vi "main.vi"() -> ()   [LabVIEW 2018]
uses:
  <vilib>/Platform/TimedLoop/XDataNode/timing_clust.ctl
  <vilib>/Platform/TimedLoop/XDataNode/nitl_modes.ctl
  <vilib>/Platform/TimedLoop/XDataNode/wakeup.ctl
  <vilib>/FPGAPlugInAG/PCIe-7841R/niLvFpga_Open_PCIe-7841R.vi
  <vilib>/rvi/interface/common/dynamic/niFpgaDynamicAddResources.vi
  <vilib>/Utility/error.llb/Error Cluster From Error Code.vi
  <vilib>/rvi/errors/niLvFpgaAdjustHostInterfaceError.vi
  <vilib>/FPGAPlugInAG/Dynamic/niLvFpga_Close_Dynamic.vi
  <vilib>/rvi/interface/nirviOpenFPGA/nirviOpenFPGA.xnode
  FPGA Bitfiles/DentalRobotEther_FPGATarget_FPGA_Y1u8jArW7bo.lvbitx
  FPGA/FPGA.vi
  <vilib>/rvi/interface/nirviReadWriteControl/nirviReadWriteControl.xnode
  <vilib>/Platform/TimedLoop/XDataNode/XDataNode.xnode
  <vilib>/rvi/interface/nirviCloseFPGA/nirviCloseFPGA.xnode
  <vilib>/Platform/TimedLoop/XDataNode/XDNodeRunTimeDep.lvlib
  <vilib>/rvi/interface/Simulation/niFpgaSimulationCallBeginRW.vi
  NiFpgaLv.dll
panel:
  in  "Tab Control 2":enum32{"Setting", "OTR", "Velocity Control"}(tab)
  in  "DC":fxp<+,32,0>=0.6999999999534339
  in  "Count/revolution":i32=17408
  in  "PID":cluster{"Kp":dbl, "Kd":dbl, "Ki":dbl}={"Kp"=0.002, "Kd"=0.007, "Ki"=9e-05}
  in  "limit_mA":dbl=480.0
  in  "inverse(degree)":i32=270
  out "Voltage Detection (mV)":cluster{dbl, "limit_mA":dbl}(graph)
  in  "DIR4":bool=TRUE
  in  "OTR":bool=TRUE
  in  "Clear":bool
  out "Inverse Count":i32
  in  "Desired RPM":dbl=200.0 step=10.0 format="%.1f"
  in  "VelCtrl":bool=TRUE
  out "Finished Late_Current Feedback":u32
  out "Finished Late_Tool Control":u32
  out "Real RPM":dbl format="%.1f"
  out "store":fxp<+,32,0>[](array[numeric])
  in  "temp":i32
  in  "Inv":bool
  in  "wait":i32
  out "Position4":i32
  out "mV":i16
  in  "Rotate":bool=TRUE
  out "Finished Late_monitor":u32
  out "Finished Late_control":u32
  in  "Tab Control":enum32{"Joints", "Position"}(tab)
  in  "Joints":sgl[](array[numeric]) step=1 format="%#_6f"
  in  "Position":sgl[](array[numeric]) step=1 format="%#_6f"
  in  "Motion Control":T1
  out "Position":T2 {"Z_theta" format="%#_8f"; "Y_theta" format="%#_8f"; "X_theta" format="%#_8f"; "Z" format="%#_8f"; "Y" format="%#_8f"; "X" format="%#_8f"}
  out "Joints (degree)":T3 {"Axis 6" format="%#_8f"; "Axis 5" format="%#_8f"; "Axis 4" format="%#_8f"; "Axis 3" format="%#_8f"; "Axis 2" format="%#_8f"; "Axis 1" format="%#_8f"}
  out "Error code":u16
  out "Motion Status":T4
  in  "Robot Control":T5
  out "Robot status":T6
  in  "stop":bool
  # "Robot Arm Control"
  # "Tool Control"
  # "Monitor"
  # "Control Panel"
  # "Intermediate Informations"
  # "Tool Setting"
  # "OTR Setting"
  # "Current Feedback"
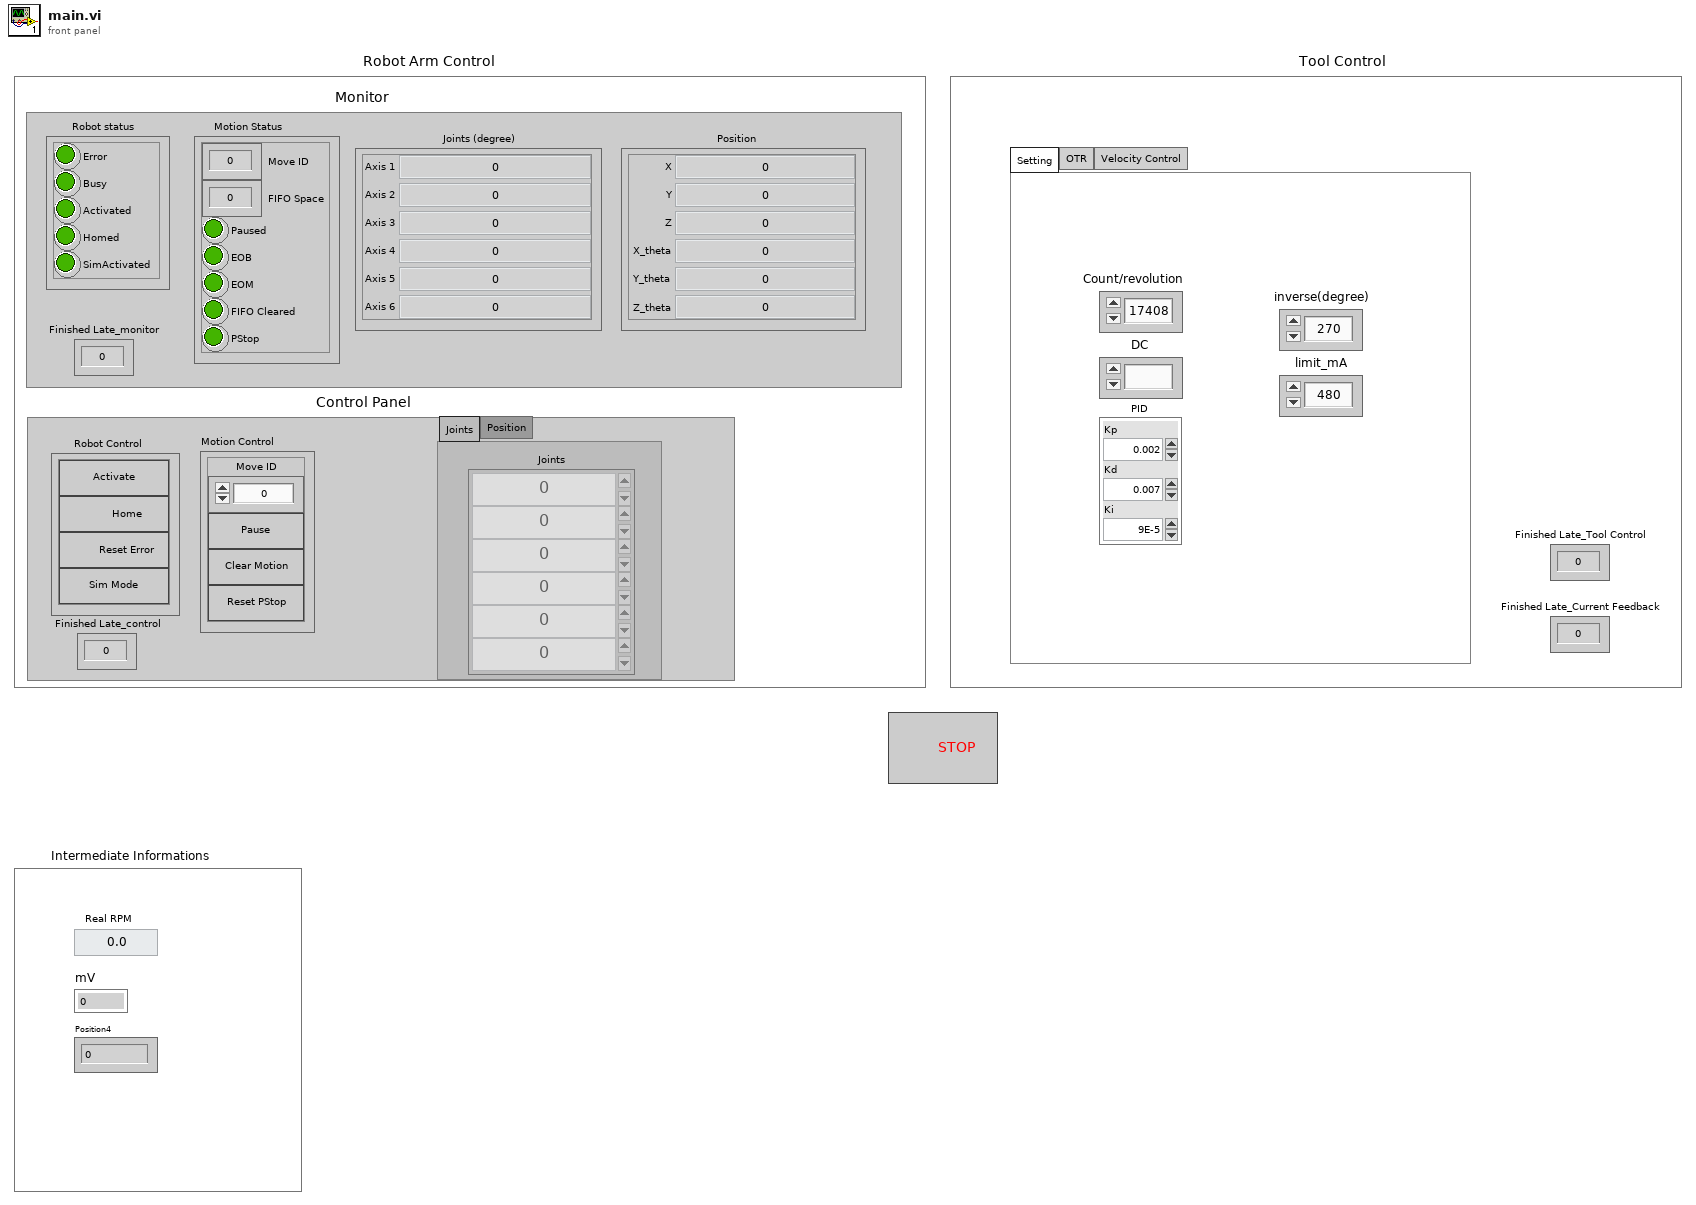
[diagram p1: front panel]
types:
  T1 = cluster{"Move ID":u16, "Pause":bool, "Clear Move":bool, "Reset PStop":bool}
  T2 = cluster{"X":sgl, "Y":sgl, "Z":sgl, "X_theta":sgl, "Y_theta":sgl, "Z_theta":sgl}
  T3 = cluster{"Axis 1":sgl, "Axis 2":sgl, "Axis 3":sgl, "Axis 4":sgl, "Axis 5":sgl, "Axis 6":sgl}
  T4 = cluster{"Move ID":dbl, "FIFO Space":dbl, "Paused":bool, "EOB":bool, "EOM":bool, "FIFO Cleared":bool, "PStop":bool}
  T5 = cluster{"Activate":bool, "Home":bool, "Reset":bool, "Sim Mode":bool}
  T6 = cluster{"Error":bool, "Busy":bool, "Activated":bool, "Homed":bool, "SimActivated":bool}
  T7 = typedef "XDNodeRunTimeDep.lvlib/timing_clust.ctl" = cluster{"Expected End [f-1]":u64, "Actual End [f-1]":u64, "Finished Late? [f-1]":bool, "Expected End [i-1]":u64, "Actual End [i-1]":u64, "Finished Late? [i-1]":bool, "Expected Start [i]":u64, "Actual Start [i]":u64, "Expected Start [f]":u64, "Actual Start [f]":u64, "Source Name":string, "Structure Name":string, "Period":i64, "Deadline":i64, "Offset":i64, "Start":i64, "Priority":i32, "Timeout":i32, "Mode":T8, "Wakeup Reason":T9, "Error":errorcluster, "Source Type":string, "Secondary Source Type":string, "Global End Time":u64, "Global Start Time":u64, "Frame Duration":u64, "Iteration Duration":u64, "Assigned CPU":i32, "I/O Scan Engine Mode":u32}
  T8 = typedef "XDNodeRunTimeDep.lvlib/nitl_modes.ctl" = enum32{"No Change", "Process missed periods, maintain original phase", "Discard missed periods, maintain original phase", "Process missed periods, ignore original phase", "Discard missed periods, ignore original phase"}
  T9 = typedef "XDNodeRunTimeDep.lvlib/wakeup.ctl" = enum32{"Normal", "Aborted", "Asynchronous wakeup", "Timing source error", "Timed loop error", "Timeout"}
  T10 = cluster{"Connector0/AI0":i16, "Connector0/AI1":i16, "Connector0/AI2":i16, "Connector0/AI3":i16, "Connector0/AI4":i16}
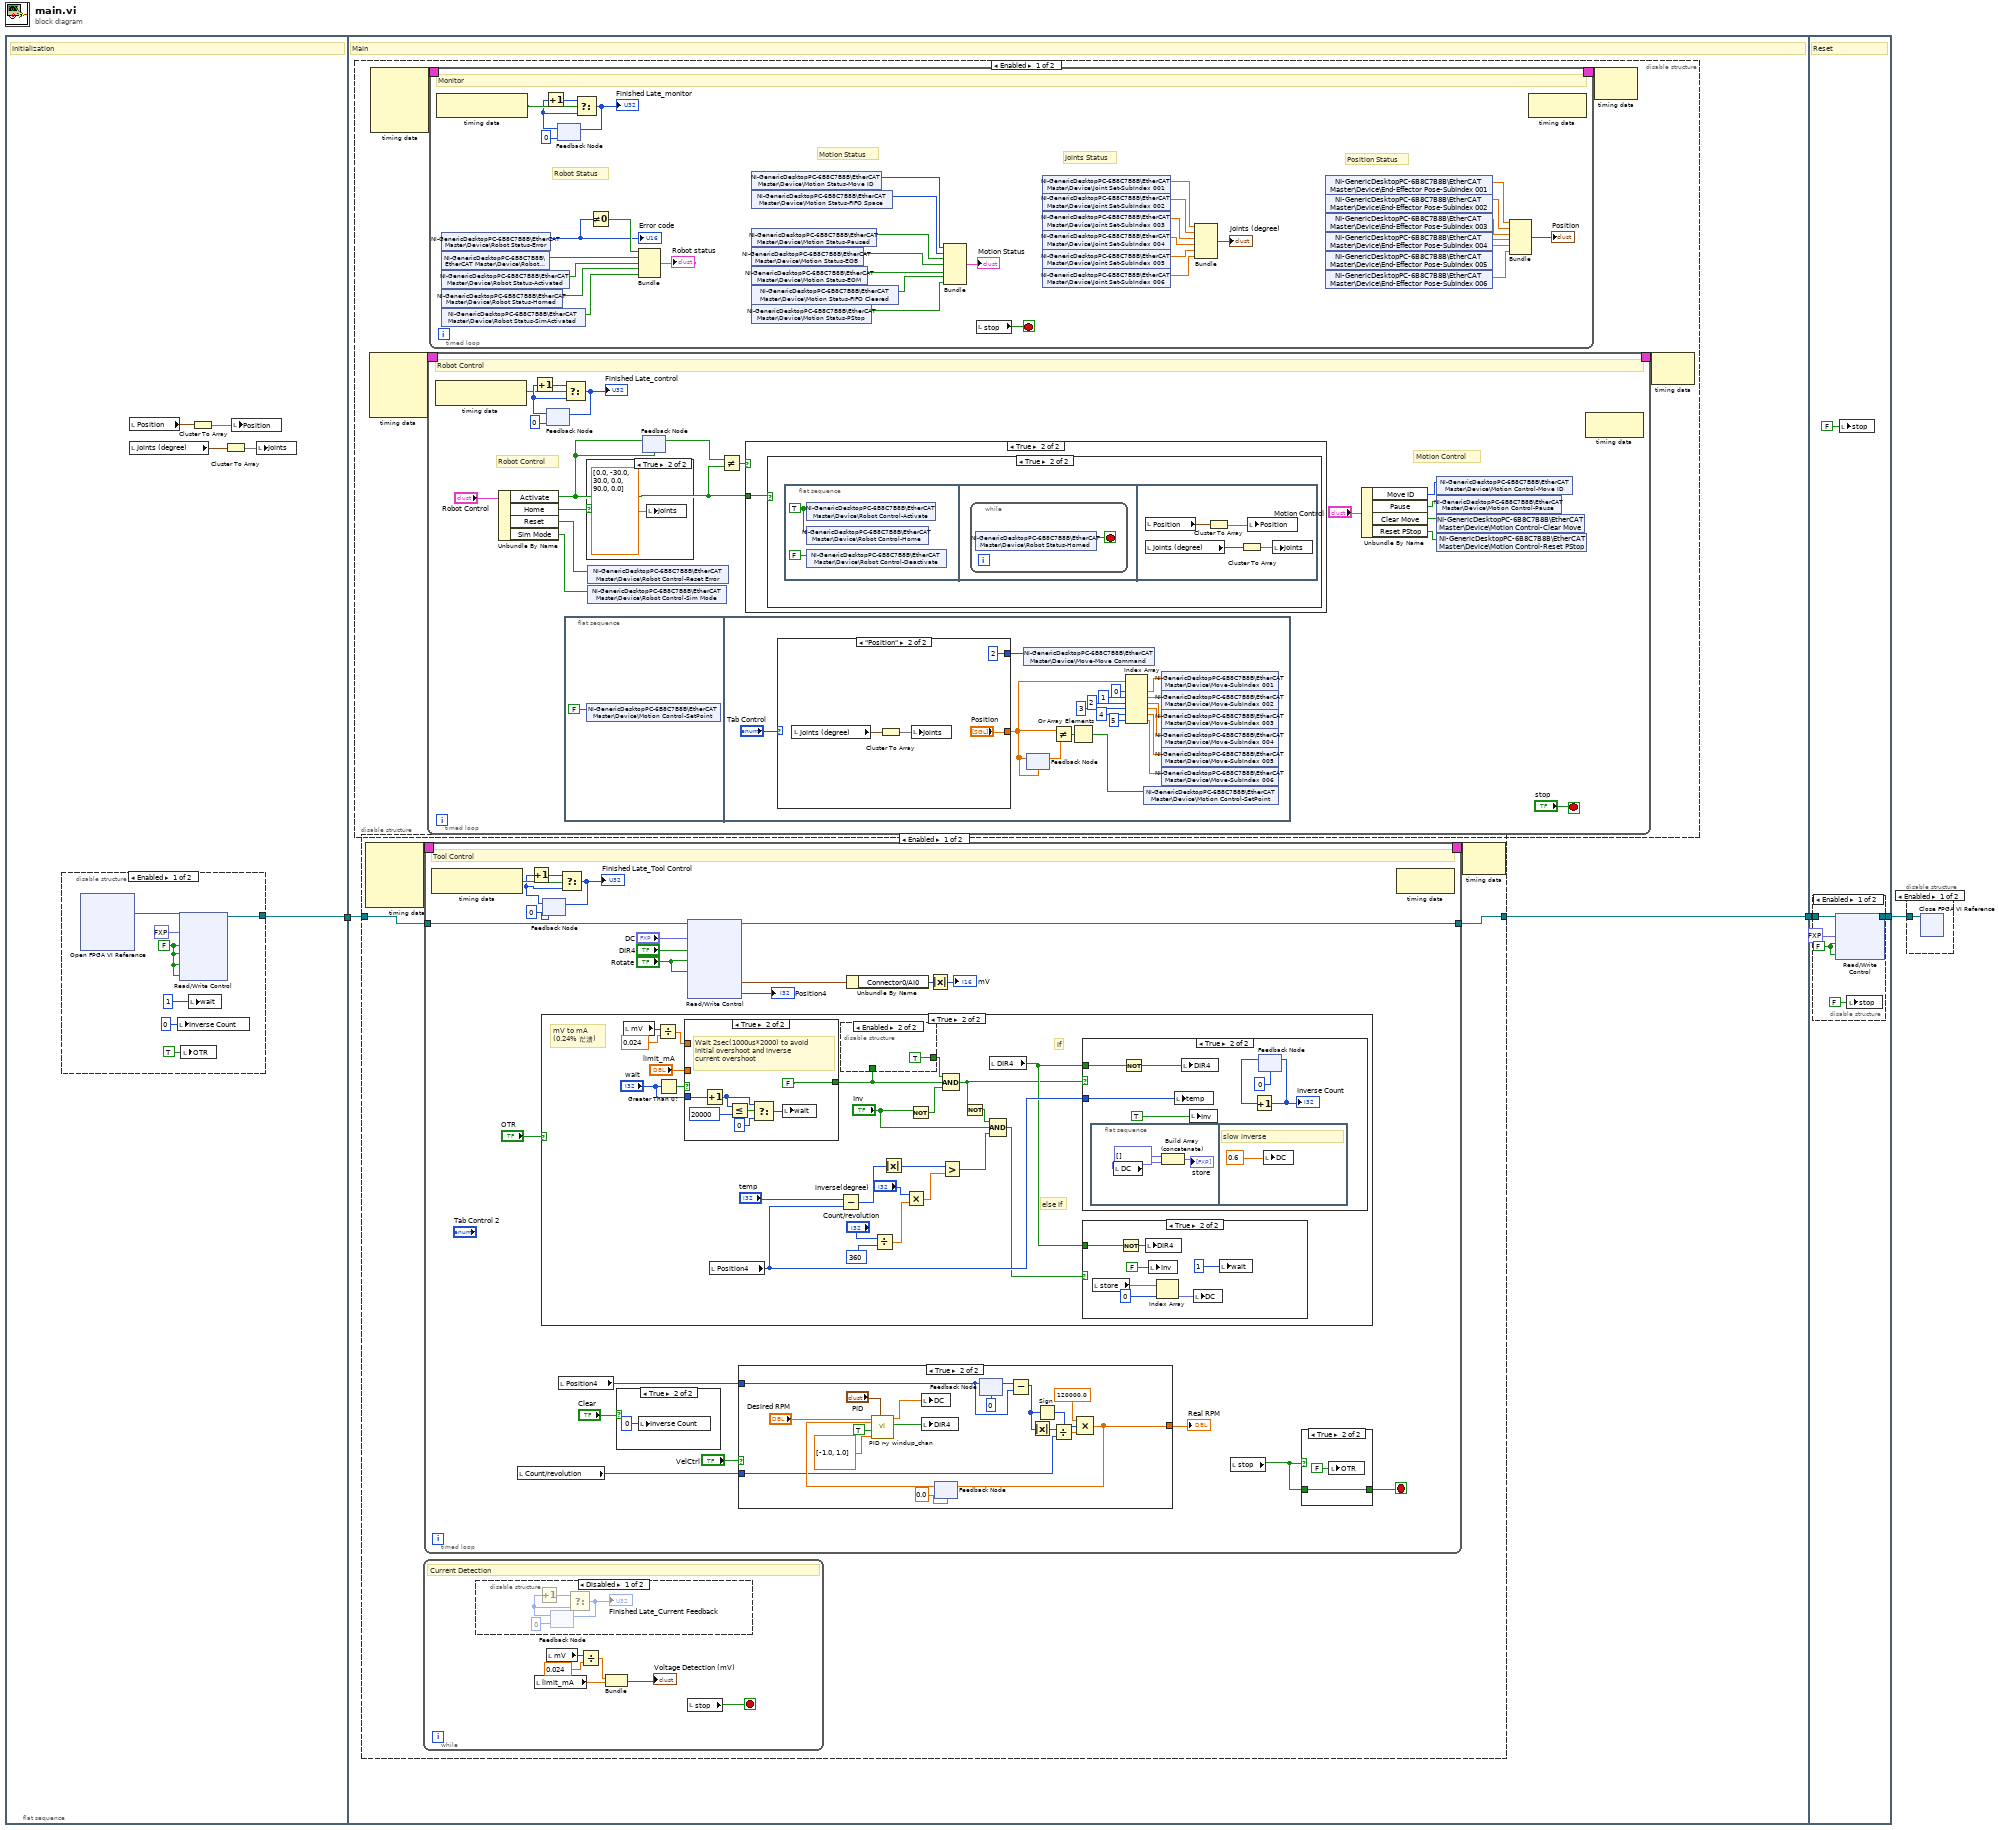
[diagram p0: block diagram]
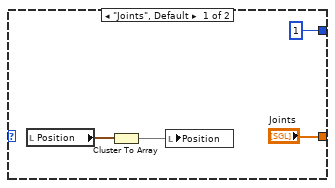
[diagram p4: hidden frame]
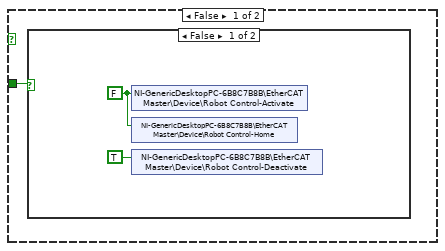
[diagram p5: hidden frame]
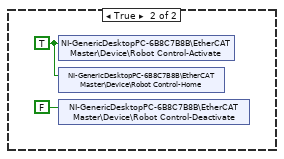
[diagram p6: hidden frame]
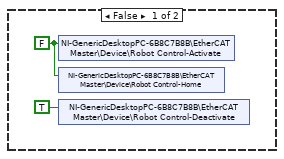
[diagram p7: hidden frame]
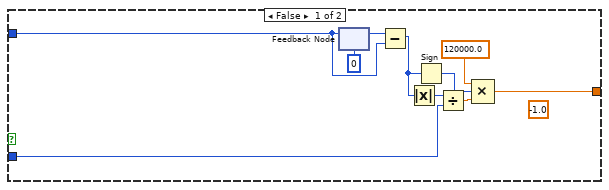
[diagram p13: hidden frame]
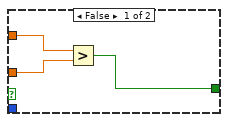
[diagram p15: hidden frame]
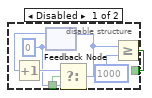
[diagram p16: hidden frame]
diagram:
  n1 = flat-sequence {
    tunnel: [w8] -> w3
    tunnel: w3 -> [w17]
    tunnel: [w16] -> w2
    tunnel: w2 -> [w263]
    tunnel: [w262] -> w1
    frame #0 {
      # "Initialization"
      n2 = disable-structure shown="Enabled" {
        disable-tunnel: [w15 _] -> w8
        frame Enabled {
          w13 = FALSE ("Reset4")
          n3 = xnode "Open FPGA VI Reference"() -> ("FPGA VI Reference Out"=w9:refnum<k20>)  [unwired: 2 in, 1 out]
          n4 = local write "Inverse Count"(0 ("Inverse Count")) -> ()
          n5 = xnode "Read/Write Control"("FPGA VI Reference In"=w9, "CH4 DC"=fxp<+,32,0> 0.0, "Reset4"=w13, "STBY4"=w13, "ENA4"=w13, "DIR4"=w13) -> ("FPGA VI Reference Out"=w15:refnum<k20>)  [unwired: 1 in, 1 out]
          n6 = local write "OTR"(TRUE ("OTR")) -> ()
          n7 = local write "wait"(1 ("wait")) -> ()
        }
        frame Disabled {
        }
      }
      n8 = local read "Position"() -> (w6:T2)
      n9 = local read "Joints (degree)"() -> (w4:T3)
      n10 = Cluster To Array(cluster=w6) -> (array=w7:sgl[])
      n11 = Cluster To Array(cluster=w4) -> (array=w5:sgl[])
      n12 = local write "Position"(w7) -> ()
      n13 = local write "Joints"(w5) -> ()
    }
    frame #1 {
      # "Main"
      n14 = disable-structure shown="Enabled" {
        frame Enabled {
          n15 = node-c288() -> (w21:T7)  [unwired: 4 in]
          n16 = node-c288() -> (w19:T7)  [unwired: 4 in]
          n17 = timed-loop {
            timing: w21 -> [_]
            timing-out: [_] -> w20
            stop <- "stop" stop-if-true
            # "Motion Control"
            # "Robot Control"
            # "Robot Control"
            n18 = node-c288() -> (w66:bool)  [unwired: 1 in]
            n19 = Unbundle By Name("Robot Control") -> ("Activate"=w63:bool, "Home"=w77:bool, "Reset"=w76:bool, "Sim Mode"=w75:bool)
            n20 = feedback #1(u32 0) -> (w68:u32)
            n21 = Increment(x=w68) -> (x+1=w69:u32)
            n22 = Select(t=w69, s=w66, f=w68) -> (s? t:f=w65:u32)
            "Finished Late_control" <- w65
            n23 = feedback-in #1(w65) -> ()
            n24 = flat-sequence {
              frame #0 {
                n25 = shared-variable "NI-GenericDesktopPC-6B8C7B8B\\EtherCAT Master\\Device\\Motion Control-SetPoint"(FALSE ("Motion Control-SetPoint")) -> ()  [unwired: 1 in, 1 out]
              }
              frame #1 {
                n26 = case shown="\"Position\"" "Tab Control" {
                  tunnel: [u32 1 ("Move-Move Command") u32 2 ("Move-Move Command")] -> w88
                  tunnel: ["Joints" "Position"] -> w87
                  frame "Joints", Default {
                    n27 = local read "Position"() -> (w100:T2)
                    n28 = Cluster To Array(cluster=w100) -> (array=w99:sgl[])
                    n29 = local write "Position"(w99) -> ()
                  }
                  frame "Position" {
                    n30 = local read "Joints (degree)"() -> (w105:T3)
                    n31 = Cluster To Array(cluster=w105) -> (array=w104:sgl[])
                    n32 = local write "Joints"(w104) -> ()
                  }
                }
                n33 = shared-variable "NI-GenericDesktopPC-6B8C7B8B\\EtherCAT Master\\Device\\Move-Move Command"(w88) -> ()  [unwired: 1 in, 1 out]
                n34 = feedback #2(w87) -> (w98:sgl[])
                n35 = feedback-in #2(w87) -> ()
                n36 = Not Equal?(x=w87, y=w98) -> (x != y?=w97:bool[])
                n37 = Or Array Elements(Boolean array=w97) -> (logical OR=w90:bool)
                n38 = Index Array(array=w87, index #1=0 ("index"), index #2=1 ("index"), index #3=2 ("index"), index #4=3 ("index"), index #5=4 ("index"), index #6=5 ("index")) -> (element #1=w86:sgl, element #2=w85:sgl, element #3=w84:sgl, element #4=w83:sgl, element #5=w82:sgl, element #6=w81:sgl)
                n39 = shared-variable "NI-GenericDesktopPC-6B8C7B8B\\EtherCAT Master\\Device\\Motion Control-SetPoint"(w90) -> ()  [unwired: 1 in, 1 out]
                n40 = shared-variable "NI-GenericDesktopPC-6B8C7B8B\\EtherCAT Master\\Device\\Move-SubIndex 001"(w86) -> ()  [unwired: 1 in, 1 out]
                n41 = shared-variable "NI-GenericDesktopPC-6B8C7B8B\\EtherCAT Master\\Device\\Move-SubIndex 002"(w85) -> ()  [unwired: 1 in, 1 out]
                n42 = shared-variable "NI-GenericDesktopPC-6B8C7B8B\\EtherCAT Master\\Device\\Move-SubIndex 003"(w84) -> ()  [unwired: 1 in, 1 out]
                n43 = shared-variable "NI-GenericDesktopPC-6B8C7B8B\\EtherCAT Master\\Device\\Move-SubIndex 004"(w83) -> ()  [unwired: 1 in, 1 out]
                n44 = shared-variable "NI-GenericDesktopPC-6B8C7B8B\\EtherCAT Master\\Device\\Move-SubIndex 005"(w82) -> ()  [unwired: 1 in, 1 out]
                n45 = shared-variable "NI-GenericDesktopPC-6B8C7B8B\\EtherCAT Master\\Device\\Move-SubIndex 006"(w81) -> ()  [unwired: 1 in, 1 out]
              }
            }
            n46 = case shown="True" w77 {
              frame False {
              }
              frame True {
                n47 = local write "Joints"(sgl[] [0.0, -30.0, 30.0, 0.0, 90.0, 0.0] ("Move SubIndex")) -> ()
              }
            }
            n48 = shared-variable "NI-GenericDesktopPC-6B8C7B8B\\EtherCAT Master\\Device\\Robot Control-Reset Error"(w76) -> ()  [unwired: 1 in, 1 out]
            n49 = shared-variable "NI-GenericDesktopPC-6B8C7B8B\\EtherCAT Master\\Device\\Robot Control-Sim Mode"(w75) -> ()  [unwired: 1 in, 1 out]
            n50 = feedback-in #3(w63) -> ()
            n51 = feedback #3(w63) -> (w62:bool)
            n52 = Not Equal?(x=w62, y=w63) -> (x != y?=w64:bool)
            n53 = case shown="True" w64 {
              tunnel: w63 -> [w107 w112]
              frame False {
                n54 = case shown="False" w107 {
                  frame False {
                    w108 = FALSE ("Robot Control-Activate")
                    n55 = shared-variable "NI-GenericDesktopPC-6B8C7B8B\\EtherCAT Master\\Device\\Robot Control-Activate"(w108) -> ()  [unwired: 1 in, 1 out]
                    n56 = shared-variable "NI-GenericDesktopPC-6B8C7B8B\\EtherCAT Master\\Device\\Robot Control-Home"(w108) -> ()  [unwired: 1 in, 1 out]
                    n57 = shared-variable "NI-GenericDesktopPC-6B8C7B8B\\EtherCAT Master\\Device\\Robot Control-Deactivate"(TRUE ("Robot Control-Deactivate")) -> ()  [unwired: 1 in, 1 out]
                  }
                  frame True {
                    w111 = TRUE ("Robot Control-Activate")
                    n58 = shared-variable "NI-GenericDesktopPC-6B8C7B8B\\EtherCAT Master\\Device\\Robot Control-Activate"(w111) -> ()  [unwired: 1 in, 1 out]
                    n59 = shared-variable "NI-GenericDesktopPC-6B8C7B8B\\EtherCAT Master\\Device\\Robot Control-Home"(w111) -> ()  [unwired: 1 in, 1 out]
                    n60 = shared-variable "NI-GenericDesktopPC-6B8C7B8B\\EtherCAT Master\\Device\\Robot Control-Deactivate"(FALSE ("Robot Control-Deactivate")) -> ()  [unwired: 1 in, 1 out]
                  }
                }
              }
              frame True {
                n61 = case shown="True" w112 {
                  frame False {
                    w114 = FALSE ("Robot Control-Activate")
                    n62 = shared-variable "NI-GenericDesktopPC-6B8C7B8B\\EtherCAT Master\\Device\\Robot Control-Activate"(w114) -> ()  [unwired: 1 in, 1 out]
                    n63 = shared-variable "NI-GenericDesktopPC-6B8C7B8B\\EtherCAT Master\\Device\\Robot Control-Home"(w114) -> ()  [unwired: 1 in, 1 out]
                    n64 = shared-variable "NI-GenericDesktopPC-6B8C7B8B\\EtherCAT Master\\Device\\Robot Control-Deactivate"(TRUE ("Robot Control-Deactivate")) -> ()  [unwired: 1 in, 1 out]
                  }
                  frame True {
                    n65 = flat-sequence {
                      frame #0 {
                        w116 = TRUE ("Robot Control-Activate")
                        n66 = shared-variable "NI-GenericDesktopPC-6B8C7B8B\\EtherCAT Master\\Device\\Robot Control-Activate"(w116) -> ()  [unwired: 1 in, 1 out]
                        n67 = shared-variable "NI-GenericDesktopPC-6B8C7B8B\\EtherCAT Master\\Device\\Robot Control-Home"(w116) -> ()  [unwired: 1 in, 1 out]
                        n68 = shared-variable "NI-GenericDesktopPC-6B8C7B8B\\EtherCAT Master\\Device\\Robot Control-Deactivate"(FALSE ("Robot Control-Deactivate")) -> ()  [unwired: 1 in, 1 out]
                      }
                      frame #1 {
                        n69 = while {
                          stop <- w117 stop-if-true
                          n70 = shared-variable "NI-GenericDesktopPC-6B8C7B8B\\EtherCAT Master\\Device\\Robot Status-Homed"() -> (w117:bool)  [unwired: 1 in, 1 out]
                        }
                      }
                      frame #2 {
                        n71 = local read "Position"() -> (w119:T2)
                        n72 = local read "Joints (degree)"() -> (w121:T3)
                        n73 = Cluster To Array(cluster=w119) -> (array=w118:sgl[])
                        n74 = Cluster To Array(cluster=w121) -> (array=w120:sgl[])
                        n75 = local write "Position"(w118) -> ()
                        n76 = local write "Joints"(w120) -> ()
                      }
                    }
                  }
                }
              }
            }
            n77 = Unbundle By Name("Motion Control") -> ("Move ID"=w73:u16, "Pause"=w72:bool, "Clear Move"=w71:bool, "Reset PStop"=w70:bool)
            n78 = shared-variable "NI-GenericDesktopPC-6B8C7B8B\\EtherCAT Master\\Device\\Motion Control-Move ID"(w73) -> ()  [unwired: 1 in, 1 out]
            n79 = shared-variable "NI-GenericDesktopPC-6B8C7B8B\\EtherCAT Master\\Device\\Motion Control-Pause"(w72) -> ()  [unwired: 1 in, 1 out]
            n80 = shared-variable "NI-GenericDesktopPC-6B8C7B8B\\EtherCAT Master\\Device\\Motion Control-Clear Move"(w71) -> ()  [unwired: 1 in, 1 out]
            n81 = shared-variable "NI-GenericDesktopPC-6B8C7B8B\\EtherCAT Master\\Device\\Motion Control-Reset PStop"(w70) -> ()  [unwired: 1 in, 1 out]
            n82 = node-c288() -> ()  [unwired: 1 in, 1 out]
          }
          n83 = timed-loop {
            timing: w19 -> [_]
            timing-out: [_] -> w18
            stop <- w44 stop-if-true
            # "Position Status"
            # "Joints Status"
            # "Motion Status"
            # "Robot Status"
            # "Monitor"
            n84 = node-c288() -> (w46:bool)  [unwired: 1 in]
            n85 = shared-variable "NI-GenericDesktopPC-6B8C7B8B\\EtherCAT Master\\Device\\Robot Status-Error"() -> (w55:u16)  [unwired: 1 in, 1 out]
            "Error code" <- w55
            n86 = shared-variable "NI-GenericDesktopPC-6B8C7B8B\\EtherCAT Master\\Device\\Robot Status-Busy"() -> (w50:bool)  [unwired: 1 in, 1 out]
            n87 = shared-variable "NI-GenericDesktopPC-6B8C7B8B\\EtherCAT Master\\Device\\Robot Status-Activated"() -> (w51:bool)  [unwired: 1 in, 1 out]
            n88 = shared-variable "NI-GenericDesktopPC-6B8C7B8B\\EtherCAT Master\\Device\\Robot Status-Homed"() -> (w52:bool)  [unwired: 1 in, 1 out]
            n89 = shared-variable "NI-GenericDesktopPC-6B8C7B8B\\EtherCAT Master\\Device\\Robot Status-SimActivated"() -> (w53:bool)  [unwired: 1 in, 1 out]
            n90 = feedback #4(u32 0) -> (w45:u32)
            n91 = Increment(x=w45) -> (x+1=w49:u32)
            n92 = Select(t=w49, s=w46, f=w45) -> (s? t:f=w47:u32)
            "Finished Late_monitor" <- w47
            n93 = feedback-in #4(w47) -> ()
            n94 = Not Equal To 0?(x=w55) -> (x != 0?=w56:bool)
            n95 = Bundle(w56, w50, w51, w52, w53) -> (→"Robot status":cluster{bool, bool, bool, bool, bool})  [unwired: 1 in]
            n96 = shared-variable "NI-GenericDesktopPC-6B8C7B8B\\EtherCAT Master\\Device\\Motion Status-Move ID"() -> (w36:u16)  [unwired: 1 in, 1 out]
            n97 = shared-variable "NI-GenericDesktopPC-6B8C7B8B\\EtherCAT Master\\Device\\Motion Status-FIFO Space"() -> (w37:u16)  [unwired: 1 in, 1 out]
            n98 = shared-variable "NI-GenericDesktopPC-6B8C7B8B\\EtherCAT Master\\Device\\Motion Status-Paused"() -> (w38:bool)  [unwired: 1 in, 1 out]
            n99 = shared-variable "NI-GenericDesktopPC-6B8C7B8B\\EtherCAT Master\\Device\\Motion Status-EOB"() -> (w39:bool)  [unwired: 1 in, 1 out]
            n100 = shared-variable "NI-GenericDesktopPC-6B8C7B8B\\EtherCAT Master\\Device\\Motion Status-EOM"() -> (w40:bool)  [unwired: 1 in, 1 out]
            n101 = shared-variable "NI-GenericDesktopPC-6B8C7B8B\\EtherCAT Master\\Device\\Motion Status-FIFO Cleared"() -> (w41:bool)  [unwired: 1 in, 1 out]
            n102 = shared-variable "NI-GenericDesktopPC-6B8C7B8B\\EtherCAT Master\\Device\\Motion Status-PStop"() -> (w42:bool)  [unwired: 1 in, 1 out]
            n103 = Bundle(w36, w37, w38, w39, w40, w41, w42) -> (→"Motion Status":cluster{u16, u16, bool, bool, bool, bool, bool})  [unwired: 1 in]
            n104 = local read "stop"() -> (w44:bool)
            n105 = shared-variable "NI-GenericDesktopPC-6B8C7B8B\\EtherCAT Master\\Device\\Joint Set-SubIndex 001"() -> (w22:sgl)  [unwired: 1 in, 1 out]
            n106 = shared-variable "NI-GenericDesktopPC-6B8C7B8B\\EtherCAT Master\\Device\\Joint Set-SubIndex 002"() -> (w23:sgl)  [unwired: 1 in, 1 out]
            n107 = shared-variable "NI-GenericDesktopPC-6B8C7B8B\\EtherCAT Master\\Device\\Joint Set-SubIndex 003"() -> (w24:sgl)  [unwired: 1 in, 1 out]
            n108 = shared-variable "NI-GenericDesktopPC-6B8C7B8B\\EtherCAT Master\\Device\\Joint Set-SubIndex 004"() -> (w25:sgl)  [unwired: 1 in, 1 out]
            n109 = shared-variable "NI-GenericDesktopPC-6B8C7B8B\\EtherCAT Master\\Device\\Joint Set-SubIndex 005"() -> (w26:sgl)  [unwired: 1 in, 1 out]
            n110 = shared-variable "NI-GenericDesktopPC-6B8C7B8B\\EtherCAT Master\\Device\\Joint Set-SubIndex 006"() -> (w27:sgl)  [unwired: 1 in, 1 out]
            n111 = Bundle(w22, w23, w24, w25, w26, w27) -> (→"Joints (degree)":cluster{sgl, sgl, sgl, sgl, sgl, sgl})  [unwired: 1 in]
            n112 = shared-variable "NI-GenericDesktopPC-6B8C7B8B\\EtherCAT Master\\Device\\End-Effector Pose-SubIndex 001"() -> (w29:sgl)  [unwired: 1 in, 1 out]
            n113 = shared-variable "NI-GenericDesktopPC-6B8C7B8B\\EtherCAT Master\\Device\\End-Effector Pose-SubIndex 002"() -> (w30:sgl)  [unwired: 1 in, 1 out]
            n114 = shared-variable "NI-GenericDesktopPC-6B8C7B8B\\EtherCAT Master\\Device\\End-Effector Pose-SubIndex 003"() -> (w31:sgl)  [unwired: 1 in, 1 out]
            n115 = shared-variable "NI-GenericDesktopPC-6B8C7B8B\\EtherCAT Master\\Device\\End-Effector Pose-SubIndex 004"() -> (w32:sgl)  [unwired: 1 in, 1 out]
            n116 = shared-variable "NI-GenericDesktopPC-6B8C7B8B\\EtherCAT Master\\Device\\End-Effector Pose-SubIndex 005"() -> (w33:sgl)  [unwired: 1 in, 1 out]
            n117 = shared-variable "NI-GenericDesktopPC-6B8C7B8B\\EtherCAT Master\\Device\\End-Effector Pose-SubIndex 006"() -> (w34:sgl)  [unwired: 1 in, 1 out]
            n118 = Bundle(w29, w30, w31, w32, w33, w34) -> (→"Position":cluster{sgl, sgl, sgl, sgl, sgl, sgl})  [unwired: 1 in]
            n119 = node-c288() -> ()  [unwired: 1 in, 1 out]
          }
          n120 = node-c288(w18) -> ()  [unwired: 1 out]
          n121 = node-c288(w20) -> ()  [unwired: 1 out]
        }
        frame Disabled {
        }
      }
      n122 = disable-structure shown="Enabled" {
        disable-tunnel: w17 -> [w129 _]
        disable-tunnel: [w128 _] -> w16
        frame Enabled {
          n123 = node-c288() -> (w131:T7)  [unwired: 4 in]
          n124 = while {
            stop <- w135 stop-if-true
            # "Current Detection"
            n125 = disable-structure shown="Disabled" {
              frame Disabled {
                n126 = feedback #5(u32 0) -> (w142:u32)
                n127 = Increment(x=w142) -> (x+1=w141:u32)
                n128 = Select(t=w141, f=w142) -> (s=w139:bool, s? t:f=w140:u32)
                "Finished Late_Current Feedback" <- w140
                n129 = feedback-in #5(w140) -> ()
              }
              frame Enabled {
              }
            }
            n130 = local read "limit_mA"() -> (w133:dbl)
            n131 = local read "mV"() -> (w136:i16)
            n132 = Divide(x=w136, y=0.024) -> (x/y=w134:dbl)
            n133 = Bundle(w134, "limit_mA"=w133) -> (→"Voltage Detection (mV)":cluster{dbl, "limit_mA":dbl})  [unwired: 1 in]
            n134 = local read "stop"() -> (w135:bool)
          }
          n135 = timed-loop {
            timing: w131 -> [_]
            timing-out: [_] -> w130
            tunnel: w129 -> [w164]
            tunnel: [w143] -> w128
            stop <- w154 stop-if-true
            # "Tool Control"
            n136 = node-c288() -> (w147:bool)  [unwired: 1 in]
            n137 = local read "Count/revolution"() -> (w156:i32)
            n138 = case shown="True" "OTR" {
              frame False {
              }
              frame True {
                # "mV to mA\n(0.24% だ溃)"
                # "else if"
                # "if"
                n139 = local read "mV"() -> (w199:i16)
                n140 = Divide(x=w199, y=0.024) -> (x/y=w198:dbl)
                n141 = Greater Than 0?(x="wait") -> (x > 0?=w201:bool)
                n142 = case shown="True" w201 {
                  tunnel: [w221 FALSE] -> w208
                  tunnel: w198 -> [w223 _]
                  tunnel: "limit_mA" -> [w222 _]
                  tunnel: "wait" -> [_ w224]
                  frame False {
                    n143 = Greater?(x=w223, y=w222) -> (0:w221:bool)
                  }
                  frame True {
                    # "Wait 2sec(1000us*2000) to avoid \ninitial overshoot and inverse \ncurrent overshoot"
                    n144 = Increment(x=w224) -> (x+1=w227:i32)
                    n145 = Less Or Equal?(x=w227, y=20000) -> (x <= y?=w226:bool)
                    n146 = Select(t=w227, s=w226, f=0) -> (s? t:f=w228:i32)
                    n147 = local write "wait"(w228) -> ()
                  }
                }
                n148 = local read "Position4"() -> (w216:i32)
                n149 = Subtract(x="temp", y=w216) -> (x-y=w218:i32)
                n150 = disable-structure shown="Enabled" {
                  disable-tunnel: w208 -> [w236 _]
                  disable-tunnel: [w232 TRUE] -> w207
                  frame Disabled {
                    w231 = 0
                    n151 = feedback #6(w231) -> (w235:i32)
                    n152 = Increment(x=w235) -> (x+1=w237:i32)
                    n153 = Select(t=w237, s=w236, f=w231) -> (s? t:f=w234:i32)
                    n154 = feedback-in #6(w234) -> ()
                    n155 = Greater Or Equal?(x=w234, y=1000) -> (x >= y?=w232:bool)
                  }
                  frame Enabled {
                  }
                }
                n156 = Divide(x="Count/revolution", y=360) -> (x/y=w210:dbl)
                n157 = Absolute Value(x=w218) -> (abs(x)=w206:i32)
                n158 = Multiply(x="inverse(degree)", y=w210) -> (x*y=w214:dbl)
                n159 = Not(x="Inv") -> (.not. x?=w220:bool)
                n160 = Greater?(x=w206, y=w214) -> (0:w204:bool)
                n161 = Compound Arithmetic op=AND(w207, w208, w220) -> (w209:bool)
                n162 = Not(x=w209) -> (.not. x?=w219:bool)
                n163 = local read "DIR4"() -> (w213:bool)
                n164 = Compound Arithmetic op=AND(w219, "Inv", w204) -> (w202:bool)
                n165 = case shown="True" w202 {
                  tunnel: w213 -> [_ w245]
                  frame False {
                  }
                  frame True {
                    n166 = local read "store"() -> (w240:fxp<+,32,0>[])
                    n167 = Not(x=w245) -> (.not. x?=w244:bool)
                    n168 = local write "DIR4"(w244) -> ()
                    n169 = local write "Inv"(FALSE ("Inv")) -> ()
                    n170 = Index Array(array=w240, index=0) -> (element=w241:fxp<+,32,0>)
                    n171 = local write "DC"(w241) -> ()
                    n172 = local write "wait"(1 ("wait")) -> ()
                  }
                }
                n173 = case shown="True" w209 {
                  tunnel: w213 -> [_ w252]
                  tunnel: w216 -> [_ w251]
                  frame False {
                  }
                  frame True {
                    n174 = flat-sequence {
                      frame #0 {
                        n175 = local read "DC"() -> (w253:fxp<+,32,0>)
                        n176 = Build Array (concatenate)(fxp<+,1,1>[] [], w253) -> (→"store":fxp<+,32,0>[])
                      }
                      frame #1 {
                        # "slow inverse"
                        n177 = local write "DC"(0.6) -> ()
                      }
                    }
                    n178 = Not(x=w252) -> (.not. x?=w250:bool)
                    n179 = local write "temp"(w251) -> ()
                    n180 = local write "DIR4"(w250) -> ()
                    n181 = local write "Inv"(TRUE ("Inv")) -> ()
                    n182 = feedback #7(0) -> (w247:i32)
                    n183 = Increment(x=w247) -> (x+1=w246:i32)
                    "Inverse Count" <- w246
                    n184 = feedback-in #7(w246) -> ()
                  }
                }
              }
            }
            n185 = feedback #8(u32 0) -> (w146:u32)
            n186 = Increment(x=w146) -> (x+1=w148:u32)
            n187 = local read "Position4"() -> (w157:i32)
            n188 = Select(t=w148, s=w147, f=w146) -> (s? t:f=w149:u32)
            "Finished Late_Tool Control" <- w149
            n189 = feedback-in #8(w149) -> ()
            n190 = case shown="True" "Clear" {
              frame False {
              }
              frame True {
                n191 = local write "Inverse Count"(0 ("Inverse Count")) -> ()
              }
            }
            n192 = xnode "Read/Write Control"("FPGA VI Reference In"=w164, "CH4 DC"="DC", "DIR4"="DIR4", "STBY4"="Rotate", "ENA4"="Rotate") -> ("FPGA VI Reference Out"=w143:refnum<k20>, "Analog"=w160:T10, "Position 4"=→"Position4":i32)  [unwired: 1 in, 1 out]
            n193 = case shown="True" "VelCtrl" {
              tunnel: w157 -> [w171 w182]
              tunnel: w156 -> [w170 w181]
              tunnel: [w169 w180] -> w155
              frame False {
                (unwired) -1.0 ("value")
                n194 = feedback #9(0 ("Position4")) -> (w177:i32)
                n195 = feedback-in #9(w171) -> ()
                n196 = Subtract(x=w177, y=w171) -> (x-y=w174:i32)
                n197 = Absolute Value(x=w174) -> (abs(x)=w175:i32)
                n198 = Sign(1:w174) -> (0:w173:i32)
                n199 = Divide(x=w175, y=w170) -> (x/y=w178:dbl)
                n200 = Compound Arithmetic op=MULTIPLY(120000.0 ("x"), w173, w178) -> (w169:dbl)
              }
              frame True {
                n201 = feedback #10(0.0) -> (w186:dbl)
                n202 = call "PID r-y windup_chan.vi"("PID Gains"="PID", "Saturation"=dbl[] [-1.0, 1.0], "Reverse Motor?"=TRUE, "Encoder position"=w186, "Reference"="Desired RPM") -> ("DIR"=w184:bool, "Duty Cycle (Abs)"=w183:dbl)  [unwired: 3 in, 2 out]
                n203 = local write "DC"(w183) -> ()
                n204 = local write "DIR4"(w184) -> ()
                n205 = feedback #11(0 ("Position4")) -> (w190:i32)
                n206 = feedback-in #11(w182) -> ()
                n207 = Subtract(x=w190, y=w182) -> (x-y=w194:i32)
                n208 = Absolute Value(x=w194) -> (abs(x)=w193:i32)
                n209 = Sign(1:w194) -> (0:w195:i32)
                n210 = Divide(x=w193, y=w181) -> (x/y=w189:dbl)
                n211 = Compound Arithmetic op=MULTIPLY(120000.0 ("x"), w195, w189) -> (w180:dbl)
                n212 = feedback-in #10(w180) -> ()
              }
            }
            "Real RPM" <- w155
            n213 = Unbundle By Name(w160) -> ("Connector0/AI0"=w159:i16)
            n214 = Absolute Value(x=w159) -> (abs(x)=→"mV":i16)
            n215 = local read "stop"() -> (w153:bool)
            n216 = case shown="True" w153 {
              tunnel: w153 -> [w166 w168]
              tunnel: [w166 w168] -> w154
              frame False {
              }
              frame True {
                n217 = local write "OTR"(FALSE ("OTR")) -> ()
              }
            }
            n218 = node-c288() -> ()  [unwired: 1 in, 1 out]
          }
          n219 = node-c288(w130) -> ()  [unwired: 1 out]
        }
        frame Disabled {
        }
      }
    }
    frame #2 {
      # "Reset"
      n220 = disable-structure shown="Enabled" {
        disable-tunnel: w263 -> [w269 _]
        disable-tunnel: [w268 _] -> w262
        frame Enabled {
          w266 = FALSE ("ENA4")
          n221 = xnode "Read/Write Control"("FPGA VI Reference In"=w269, "CH4 DC"=fxp<+,32,0> 0.0, "ENA4"=w266, "STBY4"=w266) -> ("FPGA VI Reference Out"=w268:refnum<k20>)  [unwired: 1 in, 1 out]
          n222 = local write "stop"(FALSE ("stop")) -> ()
        }
        frame Disabled {
        }
      }
      n223 = local write "stop"(FALSE ("stop")) -> ()
    }
  }
  n224 = disable-structure shown="Enabled" {
    disable-tunnel: w1 -> [w270 _]
    frame Enabled {
      n225 = xnode "Close FPGA VI Reference"("FPGA VI Reference In"=w270) -> ()  [unwired: 1 in, 1 out]
    }
    frame Disabled {
    }
  }
